vi "지진계측기(교수님 코드).vi"() -> ()   [LabVIEW 2021]
uses:
  <vilib>/DAQmx/read.llb/DAQmx Read (Analog 1D DBL 1Chan NSamp).vi
  <vilib>/Analysis/baseanly.llb/Mean (DBL).vi
  <vilib>/DAQmx/create/channels.llb/DAQmx Create Channel (AI-Voltage-Basic).vi
  <vilib>/DAQmx/configure/timing.llb/DAQmx Timing (Sample Clock).vi
  <vilib>/DAQmx/miscellaneous.llb/DAQmx Fill In Error Info.vi
  <vilib>/Analysis/NI_AALBase.lvlib
panel:
  out "문자열":string
  in  "알람리셋":bool
  out "알람발생":bool
  in  "정지":bool
  in  "시작":bool
  out "웨이브폼 차트":dbl(graph)
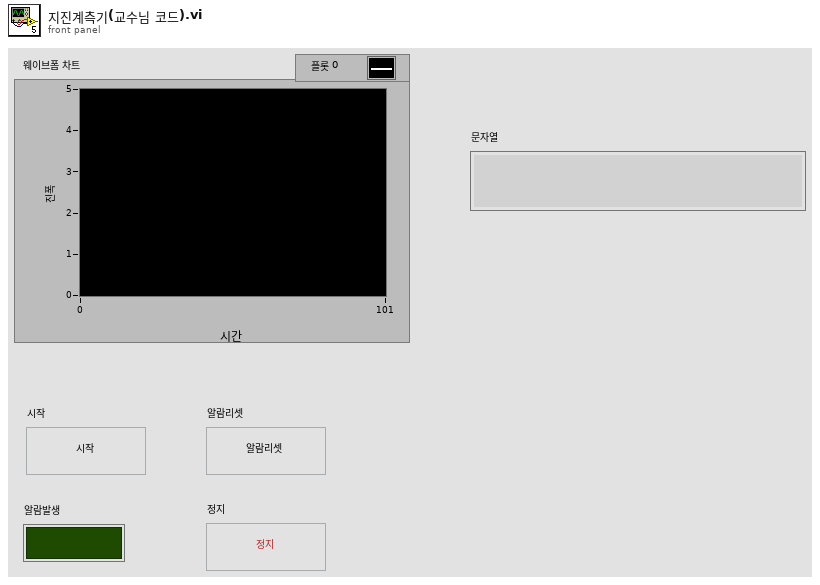
[diagram p1: front panel]
types:
  T1 = enum16{"초기화", "대기", "감지 시작", "알람 발생", "알람 리셋", "정지"}
  T2 = cluster{"task out":refnum<k21>, "알람 발생":bool, "데이터":dbl, "알람 데이터":string}
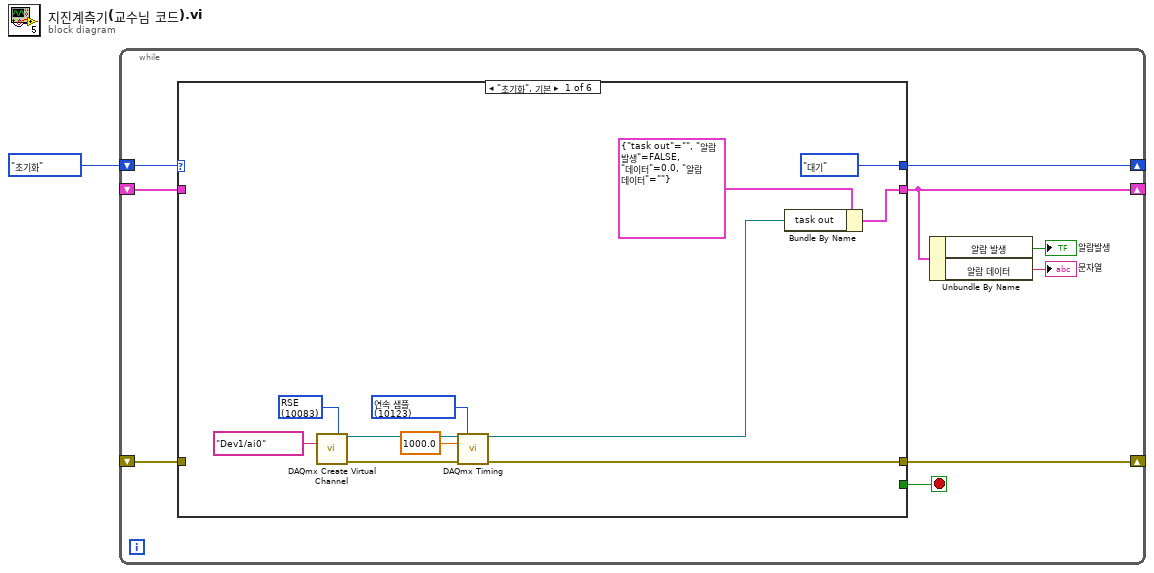
[diagram p0: block diagram]
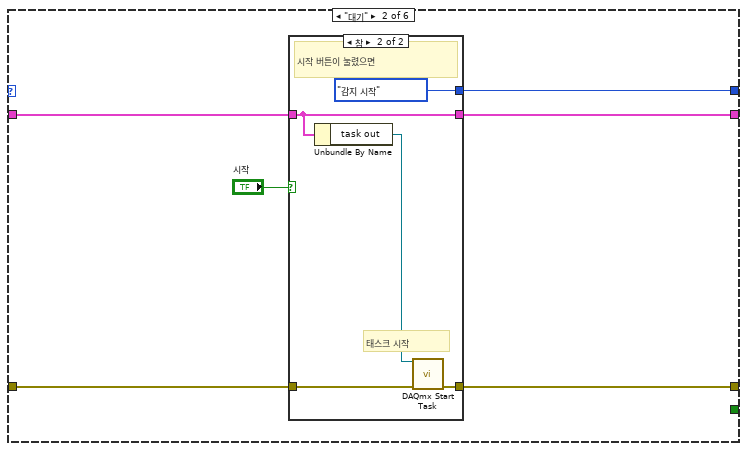
[diagram p2: hidden frame]
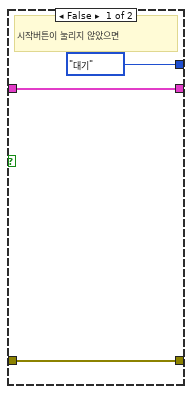
[diagram p3: hidden frame]
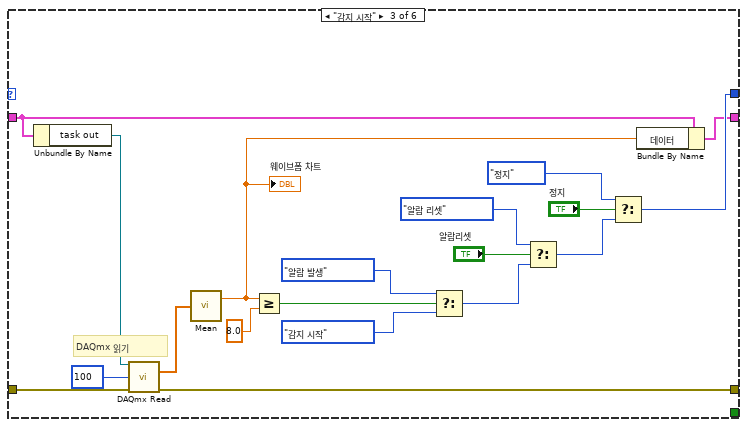
[diagram p4: hidden frame]
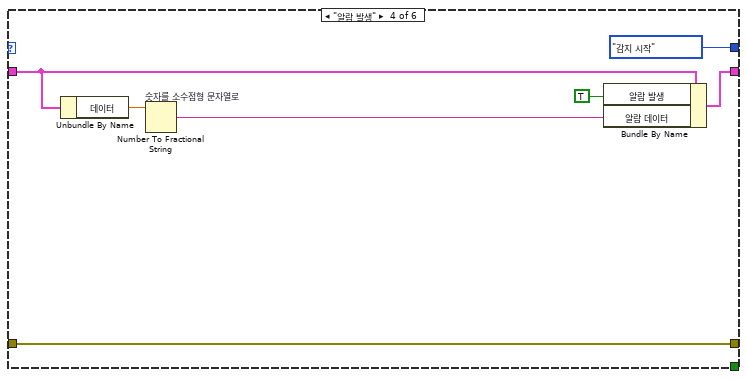
[diagram p5: hidden frame]
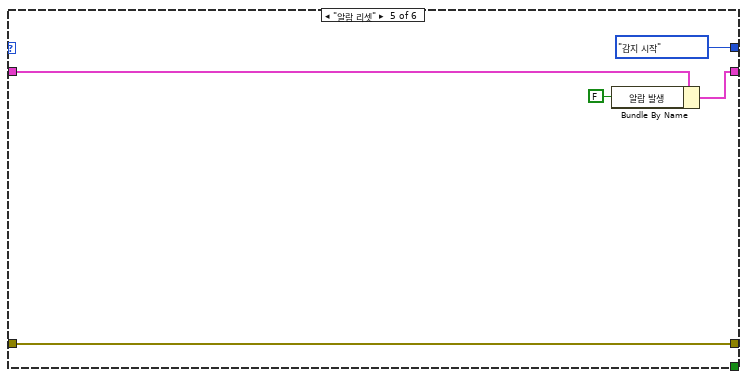
[diagram p6: hidden frame]
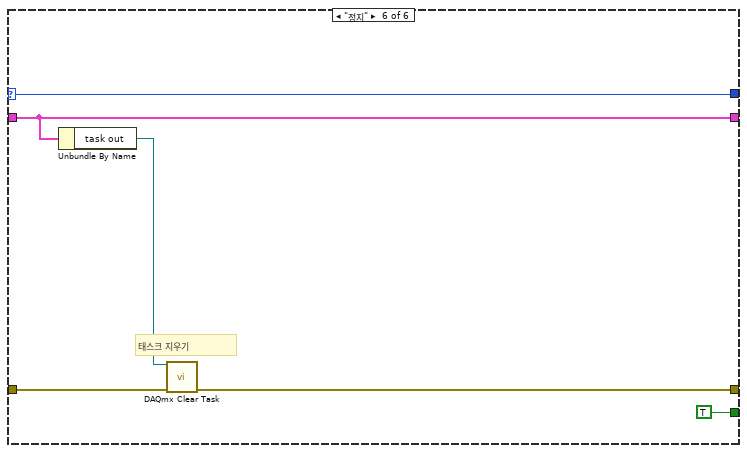
[diagram p7: hidden frame]
diagram:
  n1 = while {
    shift-right: [w9] -> _
    shift-left: T1."초기화" -> [w10]
    shift-right: [w5] -> _
    shift-left: _ -> [w8]
    shift-right: [w6] -> _
    shift-left: _ -> [w7]
    stop <- w3 stop-if-true
    n2 = case shown="\"초기화\", 기본" w10 {
      selector: w10 -> [_ _ _ _ _ w72]
      tunnel: [T1."대기" w25 w51 T1."감지 시작" T1."감지 시작" w72] -> w9
      tunnel: [w14 w23 w39 w60 w64 w71] -> w5
      tunnel: w8 -> [_ w26 w38 w57 w65 w71]
      tunnel: w7 -> [_ w24 w50 w58 w62 w70]
      tunnel: [w12 w22 w43 w58 w62 w68] -> w6
      tunnel: [_ _ _ _ _ TRUE] -> w3
      frame "초기화", Default {
        w17 = 10123 items=["유한 샘플"=10178, "연속 샘플"=10123, "하드웨어 타이밍에 의한 단일 포인트"=12522] ("sample mode")
        w18 = 10083 items=["기본"=-1, "RSE"=10083, "NRSE"=10078, "차동"=10106, "유사 차동"=12529] ("input terminal configuration")
        n3 = call-poly <vilib>:"DAQmx Create Virtual Channel.vi"("input terminal configuration"=w18, "physical channels"=tag "Dev1/ai0") -> ("task out"=w21:refnum<k21>, "error out"=w20:errorcluster)  [unwired: 12 in]
        n4 = call-poly <vilib>:"DAQmx Timing.vi"("task/channels in"=w21, "sample mode"=w17, "rate"=1000.0, "error in"=w20) -> ("task out"=w13:refnum<k21>, "error out"=w12:errorcluster)  [unwired: 10 in]
        n5 = Bundle By Name(cluster=T2 {"task out"="", "알람 발생"=FALSE, "데이터"=0.0, "알람 데이터"=""}, "task out"=w13) -> (w14:T2)
      }
      frame "대기" {
        n6 = case shown="참" "시작" {
          tunnel: w26 -> [w30 w33]
          tunnel: [T1."대기" T1."감지 시작"] -> w25
          tunnel: w24 -> [w29 w35]
          tunnel: [w30 w33] -> w23
          tunnel: [w29 w31] -> w22
          frame False {
            # "시작버튼이 눌리지 않았으면"
          }
          frame True {
            # "태스크 시작"
            # "시작 버튼이 눌렸으면"
            n7 = Unbundle By Name(w33) -> ("task out"=w34:refnum<k21>)
            n8 = call <vilib>:"DAQmx Start Task.vi"("task/channels in"=w34, "error in"=w35) -> ("error out"=w31:errorcluster)  [unwired: 12 in, 1 out]
          }
        }
      }
      frame "감지 시작" {
        # "DAQmx 읽기"
        n9 = Unbundle By Name(w38) -> ("task out"=w49:refnum<k21>)
        n10 = call-poly <vilib>:"DAQmx Read.vi"("task/channels in"=w49, "number of samples per channel"=100, "error in"=w50) -> ("data"=w47:dbl[], "error out"=w43:errorcluster)  [unwired: 10 in, 1 out]
        n11 = call-poly <vilib>:"Mean.vi"("X"=w47) -> ("mean"=w37:dbl)  [unwired: 1 out]
        "웨이브폼 차트" <- w37
        n12 = Greater Or Equal?(x=w37, y=8.0) -> (x >= y?=w46:bool)
        n13 = Select(t=T1."알람 발생", s=w46, f=T1."감지 시작") -> (s? t:f=w45:T1)
        n14 = Select(t=T1."알람 리셋", s="알람리셋", f=w45) -> (s? t:f=w52:T1)
        n15 = Select(t=T1."정지", s="정지", f=w52) -> (s? t:f=w51:T1)
        n16 = Bundle By Name(cluster=w38, "데이터"=w37) -> (w39:T2)
      }
      frame "알람 발생" {
        n17 = Unbundle By Name(w57) -> ("데이터"=w56:dbl)
        n18 = Number To Fractional String "숫자를 소수점형 문자열로"(number=w56) -> (F-format string=w55:string)  [unwired: 3 in]
        n19 = Bundle By Name(cluster=w57, "알람 발생"=TRUE, "알람 데이터"=w55) -> (w60:T2)
      }
      frame "알람 리셋" {
        n20 = Bundle By Name(cluster=w65, "알람 발생"=FALSE) -> (w64:T2)
      }
      frame "정지" {
        # "태스크 지우기"
        n21 = Unbundle By Name(w71) -> ("task out"=w69:refnum<k21>)
        n22 = call <vilib>:"DAQmx Clear Task.vi"("task in"=w69, "error in"=w70) -> ("error out"=w68:errorcluster)  [unwired: 13 in]
      }
    }
    n23 = Unbundle By Name(w5) -> ("알람 발생"=→"알람발생":bool, "알람 데이터"=→"문자열":string)
  }
